vi "getAllChannels.vi"(8 "error in (no error)":errorcluster, 11 "DeviceArray in":refnum<class "DeviceArray.lvclass">) -> (0 "error out":errorcluster, 2 "ChannelArray.lvclass":refnum<class "ChannelArray.lvclass">, 3 "DeviceArray out":refnum<class "DeviceArray.lvclass">)   [LabVIEW 2009, in "Tools.lvlib" / "DatabaseHelpers.lvlib" / "DeviceArray.lvclass"]
uses:
  DeviceArray.lvclass
  ChannelArray/ChannelArray.lvclass
  DeviceArray.lvclass/DeviceArray.ctl
  device/device.lvclass
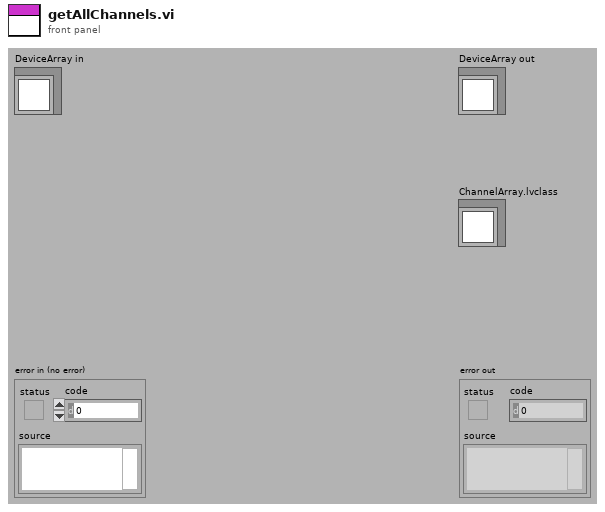
[diagram p1: front panel]
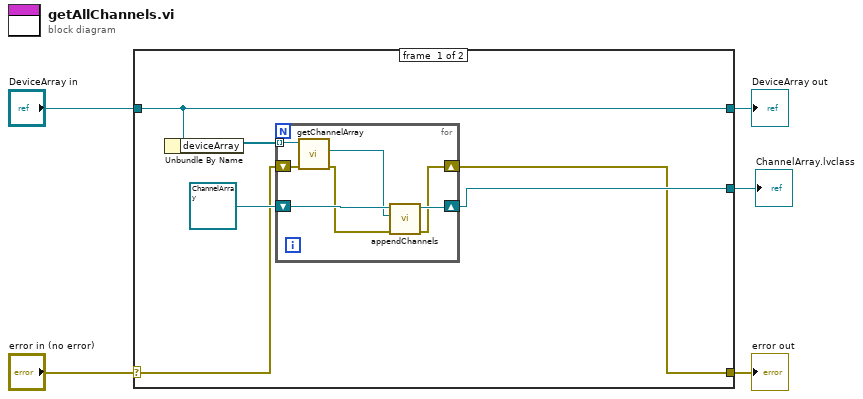
[diagram p0: block diagram]
diagram:
  n1 = case shown="No Error" "error in (no error)" {
    selector: "error in (no error)" -> [w8 w20]
    tunnel: [w6 w20] -> w4
    tunnel: [w11 w19] -> w2
    tunnel: "DeviceArray in" -> [w11 w19]
    tunnel: [w7 _] -> w1
    frame #0 {
      n2 = Unbundle By Name(w11) -> ("deviceArray"=w10:refnum<class "device.lvclass">[])
      n3 = for {
        tunnel: w10 -> [w18] mode=indexing
        shift-right: [w15] -> w7
        shift-left: refnum<class "ChannelArray.lvclass"> refnum ("ChannelArray.lvclass") -> [w17]
        shift-right: [w12] -> w6
        shift-left: w8 -> [w13]
        n4 = call "getChannelArray.vi"("error in (no error)"=w13, "device.lvclass in"=w18) -> ("error out"=w14:errorcluster, "ChannelArray.lvclass"=w16:refnum<class "ChannelArray.lvclass">)  [unwired: 7 in, 1 out]
        n5 = call "appendChannels.vi"("error in (no error)"=w14, "ChannelArrayToAppend"=w16, "ChannelArray in"=w17) -> ("error out"=w12:errorcluster, "ChannelArray out"=w15:refnum<class "ChannelArray.lvclass">)  [unwired: 7 in]
      }
    }
    frame #1 {
    }
  }
  "error out" <- w4
  "DeviceArray out" <- w2
  "ChannelArray.lvclass" <- w1
